vi "train_post.vi"(7 "LabVIEW Web Service Request":refnum<class "Web Request.lvclass">) -> ()   [LabVIEW 2014]
uses:
  <vilib>/wsapi/Web Request.lvclass
  DataManager/StateStore/Controls/DataFunction.ctl
panel:
  out "timing":u32
  out "sum":i32
  out "JSON string":string
  out "error out":errorcluster
  # "Use the Web Service Request input terminal to call the VIs on the Web Services palette. Do not remove it from the connector pane unless you don't need access to the palette."
  # "Each additional control wired to the connector pane will be available as an input in the URL. To include an indicator in terminal-mode output (the default setting), it must also be wired to the connector pane."
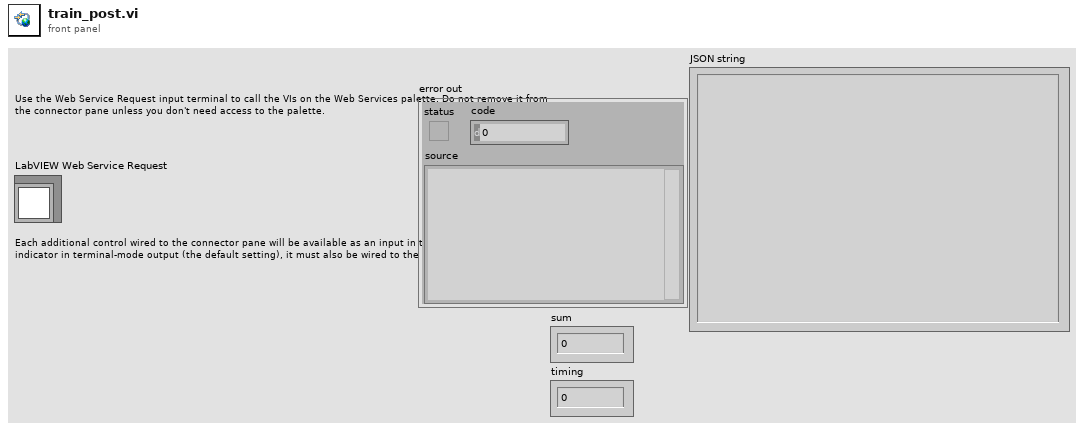
[diagram p1: front panel]
types:
  T1 = cluster{"uuid":string, "int":i32, "posit_array":cluster{"x":dbl, "y":dbl, "z":dbl}[]}[]
  T2 = typedef "DataFunction.ctl" = enum16{"Initialise", "Release", "Get Data", "Set Data", "Preview Data"}
  T3 = typedef "CData Core Control.ctl" = cluster{"train_data_array":cluster{"uuid":string, "int":i32, "posit_array":cluster{"x":dbl, "y":dbl, "z":dbl}[]}[], "train_control_array":cluster{"uuid":string, "throttle":dbl, "brake":dbl, "horn":dbl, "wait":dbl, "name":string, "mode":string, "dest":string}[], "switch_data_array":cluster{"switch_posit":cluster{"x":dbl, "y":dbl, "z":dbl}, "manual":bool}[], "switch_control_array":cluster{"switch_posit":cluster{"x":dbl, "y":dbl, "z":dbl}, "switch":bool, "invert":bool, "wait":dbl}[]}
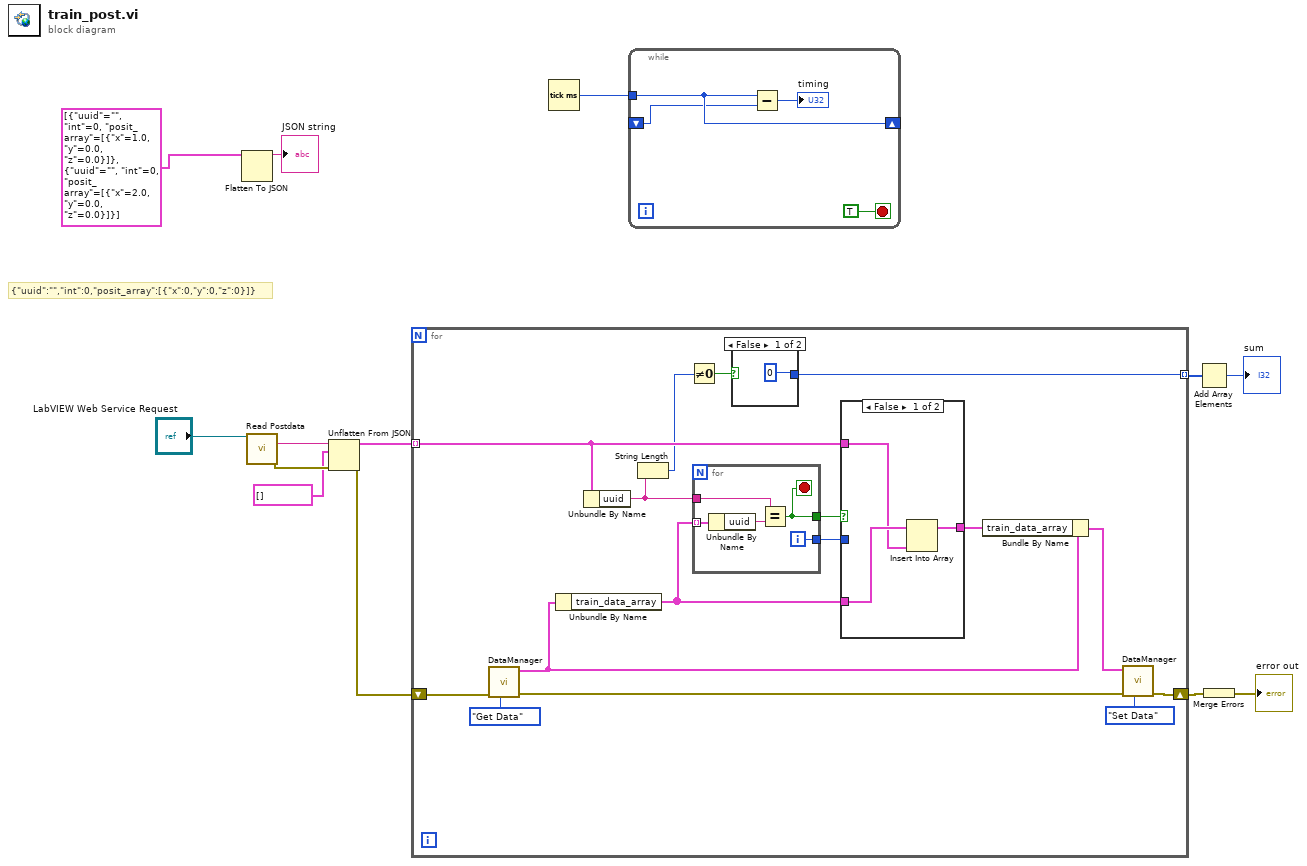
[diagram p0: block diagram]
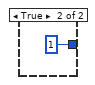
[diagram p2: hidden frame]
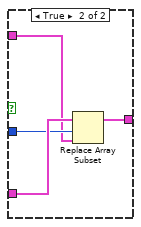
[diagram p3: hidden frame]
diagram:
  # "{\"uuid\":\"\",\"int\":0,\"posit_array\":[{\"x\":0,\"y\":0,\"z\":0}]}"
  n1 = Flatten To JSON(anything=T1 [{"uuid"="", "int"=0, "posit_array"=[{"x"=1.0, "y"=0.0, "z"=0.0}]}, {"uuid"="", "int"=0, "posit_array"=[{"x"=2.0, "y"=0.0, "z"=0.0}]}]) -> (JSON string=→"JSON string":string)  [unwired: 2 in, 1 out]
  n2 = call <vilib>:"Read Postdata.vi"("LabVIEW Web Service Request"="LabVIEW Web Service Request") -> ("postdata"=w12:string, "error out"=w8:errorcluster)  [unwired: 12 in, 1 out]
  n3 = Unflatten From JSON(JSON string=w12, type and defaults=T1 [], error in (no error)=w8) -> (value=w6:T1, error out=w9:errorcluster)  [unwired: 4 in]
  n4 = for {
    shift-right: [w21] -> w10
    shift-left: w9 -> [w19]
    tunnel: w6 -> [w18] mode=indexing
    tunnel: [w14] -> w3 mode=indexing
    n5 = call "DataManager.vi"("DataFunction"=DataFunction."Get Data", "error in (no error)"=w19) -> ("error out"=w20:errorcluster, "CData Out"=w22:T3)  [unwired: 8 in]
    n6 = Unbundle By Name(w22) -> ("train_data_array"=w24:T1)
    n7 = Unbundle By Name(w18) -> ("uuid"=w17:string)
    n8 = String Length(string=w17) -> (length=w16:i32)
    n9 = Not Equal To 0?(x=w16) -> (x != 0?=w15:bool)
    n10 = for {
      tunnel: w24 -> [w43] mode=indexing
      tunnel: w17 -> [w41]
      tunnel: [w40] -> w26
      tunnel: [w39] -> w25
      i -> [w39]
      stop <- w40 stop-if-true
      n11 = Unbundle By Name(w43) -> ("uuid"=w42:string)
      n12 = Equal?(x=w41, y=w42) -> (x = y?=w40:bool)
    }
    n13 = case shown="False" w15 {
      tunnel: [0 ("length") 1 ("length")] -> w14
      frame False {
      }
      frame True {
      }
    }
    n14 = case shown="False" w26 {
      tunnel: w25 -> [_ w37]
      tunnel: w24 -> [w34 w38]
      tunnel: w18 -> [w33 w36]
      tunnel: [w32 w35] -> w23
      frame False {
        n15 = Insert Into Array(array=w34, new element=w33) -> (w32:T1)  [unwired: 1 in]
      }
      frame True {
        n16 = Replace Array Subset(array=w38, new element=w36, index=w37) -> (w35:T1)
      }
    }
    n17 = Bundle By Name(cluster=w22, "train_data_array"=w23) -> (w27:T3)
    n18 = call "DataManager.vi"("DataFunction"=DataFunction."Set Data", "error in (no error)"=w20, "CData In"=w27) -> ("error out"=w21:errorcluster)  [unwired: 7 in, 1 out]
  }
  n19 = Tick Count (ms)() -> (millisecond timer value=w1:u32)
  n20 = while {
    tunnel: w1 -> [w47]
    shift-right: [w47] -> _
    shift-left: _ -> [w46]
    stop <- TRUE stop-if-true
    n21 = Subtract(x=w47, y=w46) -> (x-y=→"timing":u32)
  }
  n22 = Add Array Elements(numeric array=w3) -> (sum=→"sum":i32)
  n23 = Merge Errors(w10) -> (→"error out":errorcluster)
